vi "Autosort - Open file.vi"() -> (3 "Byte Stream File out":refnum<file>)   [LabVIEW 2013]
uses:
  plugins/Mars 3D/Mars3D_autosort.vi
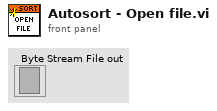
[diagram p1: front panel]
types:
  T1 = cluster{"Autosize Parameter Set 2":cluster{"Trigger Ch":i32, "Min Vel":dbl, "MaxVel":dbl, "Width":i32, "Pre Impuls":i32, "Post Impuls":i32, "Pitch":dbl, "Name":string, "Other Trigger":bool, "Cross Corr":bool, "Default":cluster{"Freq":dbl, "Vel":dbl, "Acc":dbl, "Stimulus":string}}[]}[]
  T2 = enum16{"open", "replace", "create", "open or create", "replace or create", "replace or create with confirmation"}
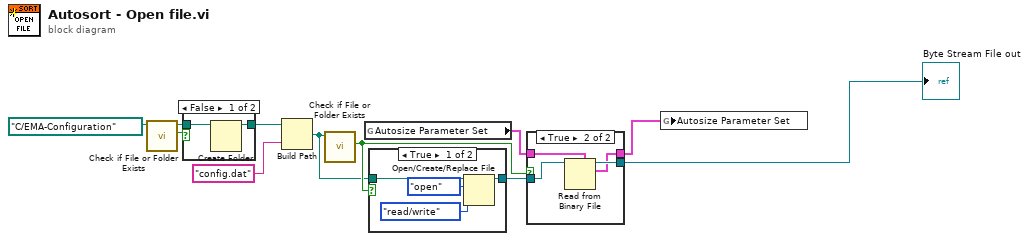
[diagram p0: block diagram]
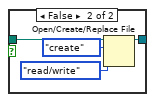
[diagram p2: hidden frame]
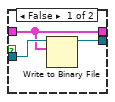
[diagram p3: hidden frame]
diagram:
  n1 = call <vilib>:"Check if File or Folder Exists.vi"("path"=path "C:/EMA-Configuration") -> ("file or folder exists?"=w6:bool, "dup path"=w7:path)  [unwired: 8 in, 1 out]
  n2 = case shown="False" w6 {
    tunnel: w7 -> [w13 w14]
    tunnel: [w12 w14] -> w8
    frame False {
      n3 = Create Folder(path (use dialog)=w13) -> (created path=w12:path)  [unwired: 2 in, 2 out]
    }
    frame True {
    }
  }
  n4 = Build Path(base path=w8, name or relative path="config.dat") -> (appended path=w10:path)
  n5 = call <vilib>:"Check if File or Folder Exists.vi"("path"=w10) -> ("file or folder exists?"=w11:bool)  [unwired: 8 in, 2 out]
  n6 = global read "Mars3D_autosort.vi" "Autosize Parameter Set"() -> (w3:T1)
  n7 = case shown="True" w11 {
    tunnel: [w17 w21] -> w1
    tunnel: w10 -> [w15 w19]
    frame True {
      n8 = Open/Create/Replace File(file path (use dialog)=w15, operation (0:open)=T2."open", access (0:read/write)=enum16{"read/write", "read-only", "write-only"}."read/write") -> (refnum out=w17:refnum<file>)  [unwired: 3 in, 2 out]
    }
    frame False {
      n9 = Open/Create/Replace File(file path (use dialog)=w19, operation (0:open)=T2."create", access (0:read/write)=enum16{"read/write", "read-only", "write-only"}."read/write") -> (refnum out=w21:refnum<file>)  [unwired: 3 in, 2 out]
    }
  }
  n10 = case shown="True" w11 {
    tunnel: w1 -> [w25 w29]
    tunnel: [w24 w28] -> w2
    tunnel: w3 -> [w23 w27]
    tunnel: [w23 w26] -> w4
    frame False {
      n11 = Write to Binary File(file (use dialog)=w25, data=w23) -> (refnum out=w24:refnum<file>)  [unwired: 4 in, 2 out]
    }
    frame True {
      n12 = Read from Binary File(5:w27, 11:w29) -> (2:w26:T1, 3:w28:refnum<file>)  [unwired: 4 in, 2 out]
    }
  }
  "Byte Stream File out" <- w2
  n13 = global write "Mars3D_autosort.vi" "Autosize Parameter Set"(w4) -> ()
